vi "Custom table polymorphic.vi"   [LabVIEW 2019]
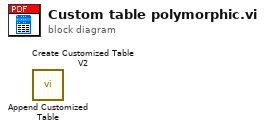
[diagram p0: block diagram]
diagram:
  n1 = call <userlib>:"Append Customized Table.vi"() -> ()  [unwired: 14 in, 2 out]
  n2 = call <vilib>:"Create Customized Table V2.vi"() -> ()  [unwired: 13 in, 3 out]
